vi "Reset Position.vi"(6 "Wait Before Reset (0ms)":u32, 7 "Position":u32, 8 "error in (no error)":errorcluster, 9 "Wait After Power On (500 ms)":u32=500, 10 "Wait After Power Off (1500 ms)":u32=1500, 11 "Driver Test":refnum<class "Driver Test.lvclass">) -> (0 "error out":errorcluster)   [LabVIEW 2015, in "Driver Test.lvclass"]
doc: "Power cycling to a position with built-in wait times for wait before power off, wait after power off, and wait after repowering."
uses:
  Driver Test.lvclass
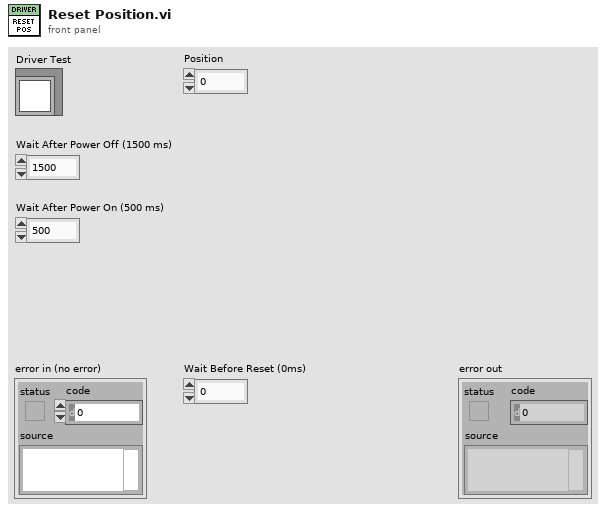
[diagram p1: front panel]
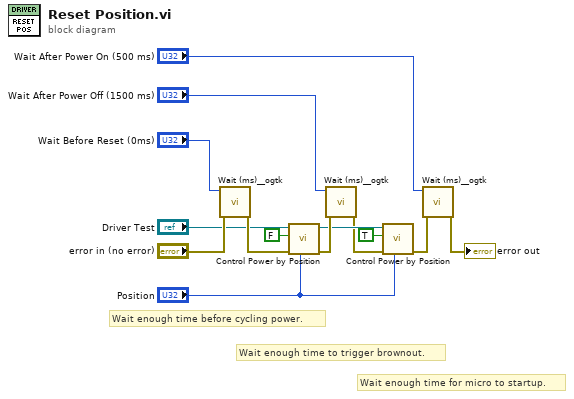
[diagram p0: block diagram]
diagram:
  # "Wait enough time for micro to startup."
  # "Wait enough time to trigger brownout."
  # "Wait enough time before cycling power."
  n1 = call <userlib>:"Wait (ms)__ogtk.vi"("error in (no error)"="error in (no error)", "milliseconds to wait"="Wait Before Reset (0ms)") -> ("error out"=w7:errorcluster)  [unwired: 8 in, 1 out]
  n2 = call "Control Power by Position.vi"("Position"="Position", "error in (no error)"=w7, "Power On?"=FALSE, "Driver Test in"="Driver Test") -> ("error out"=w6:errorcluster)  [unwired: 7 in]
  n3 = call <userlib>:"Wait (ms)__ogtk.vi"("error in (no error)"=w6, "milliseconds to wait"="Wait After Power Off (1500 ms)") -> ("error out"=w2:errorcluster)  [unwired: 8 in, 1 out]
  n4 = call "Control Power by Position.vi"("Position"="Position", "error in (no error)"=w2, "Power On?"=TRUE, "Driver Test in"="Driver Test") -> ("error out"=w1:errorcluster)  [unwired: 7 in]
  n5 = call <userlib>:"Wait (ms)__ogtk.vi"("error in (no error)"=w1, "milliseconds to wait"="Wait After Power On (500 ms)") -> ("error out"=→"error out":errorcluster)  [unwired: 8 in, 1 out]
